vi "tester.vi"() -> ()   [LabVIEW 2012, in "Retiga.lvclass"]
uses:
  Retiga.lvclass
  <vilib>/gmath/statdist.llb/st_Percentiles (scalar).vi
  <vilib>/vision/NI_Vision_Development_Module.lvlib
  <vilib>/gmath/NI_Gmath.lvlib
panel:
  out "single precision float":sgl
  in  "p":dbl
  out "Image 2":T1(plugin-control)
  in  "Settings":T2={"Objects"=1, "Threshold"=100, "Reject Border"=FALSE, "Fill Holes"=FALSE, "Min Object Size"=FALSE, "Min Size"=3, "Max Object Size"=FALSE, "Max Size"=100, "Show Search Area"=FALSE, "Show Center"=TRUE, "Show Bounding Box"=TRUE} {"Objects" items=["Bright Objects", "Dark Objects"]}
  out "Objects":T3(array[cluster]) {"Aspect Ratio" format="%.2f"; "Orientation" format="%.2f"; "Area" format="%.2f"; "Object Center"."Y" format="%.2f"; "Object Center"."X" format="%.2f"}
  out "Image":T1(plugin-control)
  in  "File Path":path
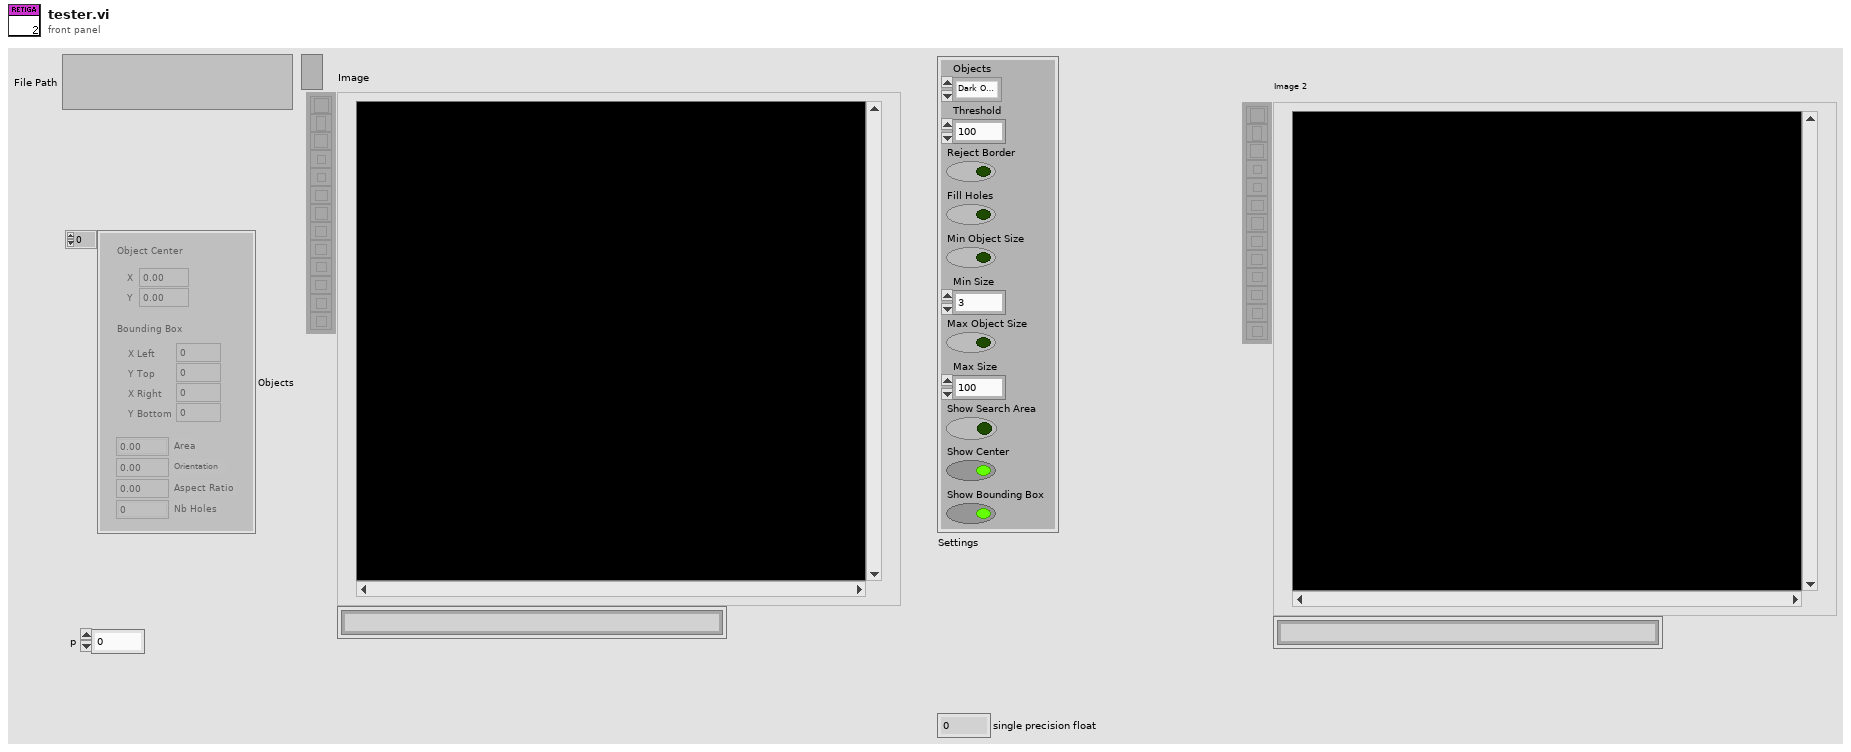
[diagram p1: front panel]
types:
  T1 = typedef "IMAQ Image.ctl" = refnum<image>
  T2 = cluster{"Objects":u16, "Threshold":i32, "Reject Border":bool, "Fill Holes":bool, "Min Object Size":bool, "Min Size":i32, "Max Object Size":bool, "Max Size":i32, "Show Search Area":bool, "Show Center":bool, "Show Bounding Box":bool}
  T3 = cluster{"Object Center":cluster{"X":sgl, "Y":sgl}, "Bounding Box":cluster{"X Left":i32, "Y Top":i32, "X Right":i32, "Y Bottom":i32}, "Area":sgl, "Orientation":sgl, "Aspect Ratio":sgl, "Nb Holes":i32}[]
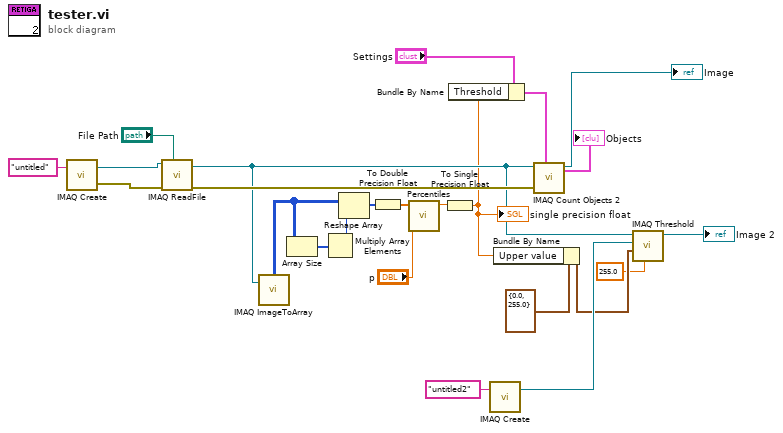
[diagram p0: block diagram]
diagram:
  n1 = call "IMAQ Create"("Image Name"="untitled") -> ("New Image"=w24:T1, "error out"=w22:errorcluster)  [unwired: 4 in]
  n2 = call "IMAQ ReadFile"("File Path"="File Path", "error in (no error)"=w22, "Image"=w24) -> ("error out"=w21:errorcluster, "Image Out"=w7:T1)  [unwired: 4 in, 3 out]
  n3 = call "IMAQ ImageToArray"("Image"=w7) -> ("Image Pixels (U8)"=w13:u8[][])  [unwired: 3 in, 4 out]
  n4 = Array Size(array=w13) -> (size(s)=w11:i32[])
  n5 = Multiply Array Elements(1:w11) -> (0:w12:i32)
  n6 = Reshape Array(w13, w12) -> (w10:u8[])
  n7 = To Double Precision Float(number=w10) -> (double precision float=w9:dbl[])
  n8 = call-poly <vilib>:"Percentiles.vi"("p"="p", "x array"=w9) -> ("percentile"=w8:dbl)  [unwired: 8 in, 1 out]
  n9 = To Single Precision Float(number=w8) -> (single precision float=w2:sgl)
  "single precision float" <- w2
  n10 = Bundle By Name(cluster="Settings", "Threshold"=w2) -> (w4:T2)
  n11 = call "IMAQ Create"("Image Name"="untitled2") -> ("New Image"=w16:T1)  [unwired: 4 in, 1 out]
  n12 = Bundle By Name(cluster=cluster{"Lower value":sgl, "Upper value":sgl} {"Lower value"=0.0, "Upper value"=255.0} ("Range"), "Upper value"=w2) -> (w3:cluster{"Lower value":sgl, "Upper value":sgl})
  n13 = call "IMAQ Count Objects 2"("Settings"=w4, "error in (no error)"=w21, "Image"=w7) -> ("Image Out"=→"Image":T1, "Objects"=→"Objects":T3)  [unwired: 4 in, 3 out]
  n14 = call "IMAQ Threshold"("Replace Value"=sgl 255.0, "Range"=w3, "Image Dst"=w16, "Image Src"=w7) -> ("Image Dst Out"=→"Image 2":T1)  [unwired: 6 in, 1 out]
